vi "DCC_get_error_string.vi"(6 "Error ID":i16, 8 "Error In":errorcluster, 11 "DLL Path":path) -> (0 "Error Out":errorcluster, 2 "Error ID":i16, 3 "DLL Path":path)   [LabVIEW 2019]
doc: "The \"DCC_get_error_string.vi\" get the corresponding error string in dependence of the given error ID.\n\nAugust 2018\nFrank Quadt & Stefan Smietana\ninfo@becker-hickl.com"
panel:
  out "Error String":string
  out "Return Type":i16
  # "(c) 2018 Becker & Hickl GmbH\n     Al Rights Reserved."
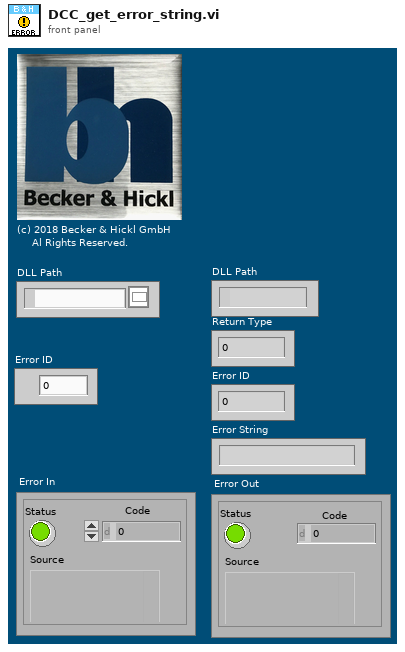
[diagram p1: front panel]
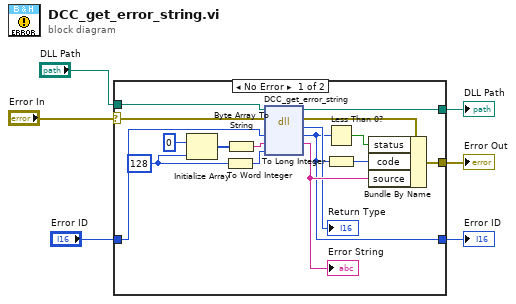
[diagram p0: block diagram]
diagram:
  n1 = case shown="No Error" "Error In" {
    selector: "Error In" -> [w22 w25]
    tunnel: [w17 w25] -> w5
    tunnel: [w21 w24] -> w4
    tunnel: "DLL Path" -> [w20 w24]
    tunnel: "Error ID" -> [w19 w23]
    tunnel: [w7 w23] -> w1
    frame No Error {
      w10 = 128 ("MaxLength")
      n2 = Initialize Array(u8 0 ("MaxLength"), w10) -> (w11:u8[])
      n3 = To Word Integer(number=w10) -> (16bit integer=w9:i16)
      n4 = Byte Array To String(unsigned byte array=w11) -> (string=w13:string)
      n5 = dll-call lib="C:/Program Files (x86)/BH/DCC/DLL/dcc64.dll" fn="DCC_get_error_string"(path in=w20, error in=w22, "ErrorID"=w19, "ErrorString"=w13, "MaxLength"=w9) -> (path out=w21:path, error out=w18:errorcluster, "return type"=→"Return Type":i16, "ErrorID"=w7:i16, "ErrorString"=w15:string)  [unwired: 2 in]
      "Error String" <- w15
      n6 = Less Than 0?(x=w7) -> (x < 0?=w16:bool)
      n7 = To Long Integer(number=w7) -> (32bit integer=w8:i32)
      n8 = Bundle By Name(cluster=w18, "status"=w16, "code"=w8, "source"=w15) -> (w17:errorcluster)
    }
    frame Error {
    }
  }
  "Error Out" <- w5
  "DLL Path" <- w4
  "Error ID" <- w1
